vi "Automatic Teller Machine (ATM).vi"() -> ()   [LabVIEW 2013]
uses:
  Controls/ATM States.ctl
  Controls/Log Data States.ctl
  SubVIs/Function Command.ctl
  Controls/Function States.ctl
panel:
  in  "Enter":bool
  in  "User Input":string
  in  "Right Buttons":T1
  out "Right Menu":T2
  in  "Left Buttons":T1
  out "Left Menu":T2
  in  "Card Simulator":bool
  out "ATM Messages":string
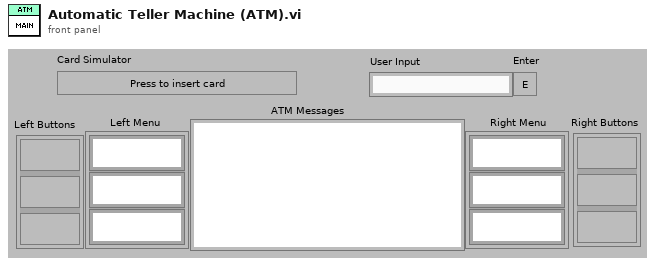
[diagram p1: front panel]
types:
  T1 = cluster{"Func Button":bool, "Func Button 2":bool, "Func Button 3":bool}
  T2 = cluster{"RFS String":string, "RFS String 2":string, "RFS String 3":string}
  T3 = cluster{"ATM Messages":string, "Left Menu":cluster{"RFS String":string, "RFS String 2":string, "RFS String 3":string}, "Right Menu":cluster{"RFS String":string, "RFS String 2":string, "RFS String 3":string}}
  T4 = typedef "ATM States.ctl" = enum16{"Initialize", "Account Check", "Main", "Withdraw", "Deposit", "Stop"}
  T5 = cluster{"Left Buttons":refnum<vi>, "Right Buttons":refnum<vi>, "Left Menu":refnum<vi>, "Right Menu":refnum<vi>, "User Input":refnum<vi>, "Enter":refnum<vi>}
  T6 = typedef "Function States.ctl" = enum16{"Check Account", "Deposit", "Withdraw"}
  T7 = typedef "Function Command.ctl" = enum16{"Set function", "Get function"}
  T8 = typedef "Log Data States.ctl" = enum16{"Initialize", "Read", "Write", "Stop"}
  T9 = enum8{"Enabled", "Disabled", "Disabled and Grayed Out"}
  T10 = cluster{"First Name":string, "Last Name":string, "Account No.":string, "Balance":i32}
  T11 = cluster{"First Name":string, "Last Name":string, "Account No.":string, "Balance":i32}[]
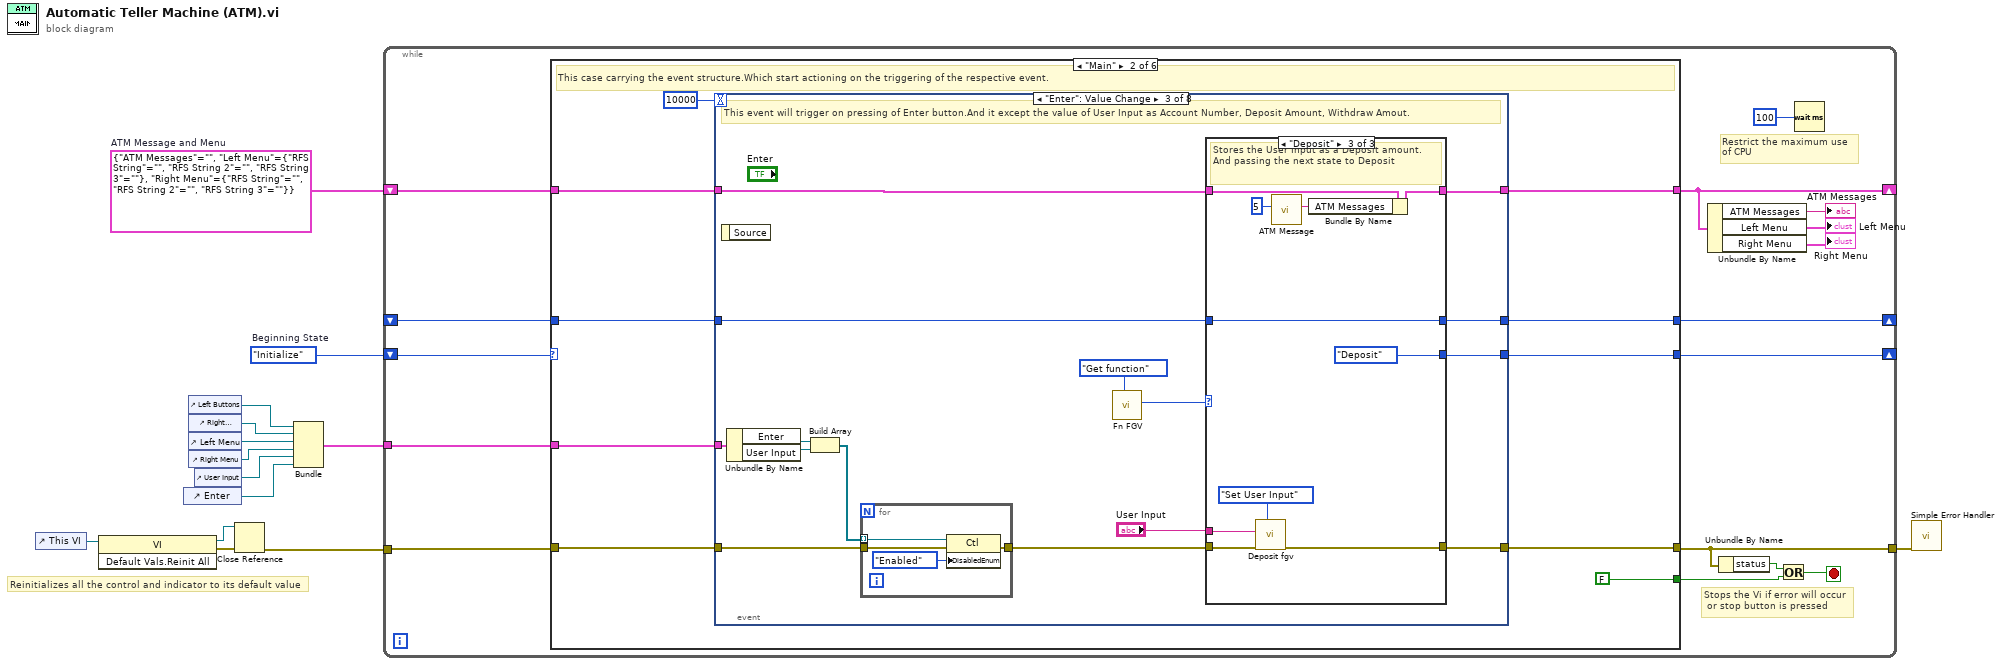
[diagram p0: block diagram]
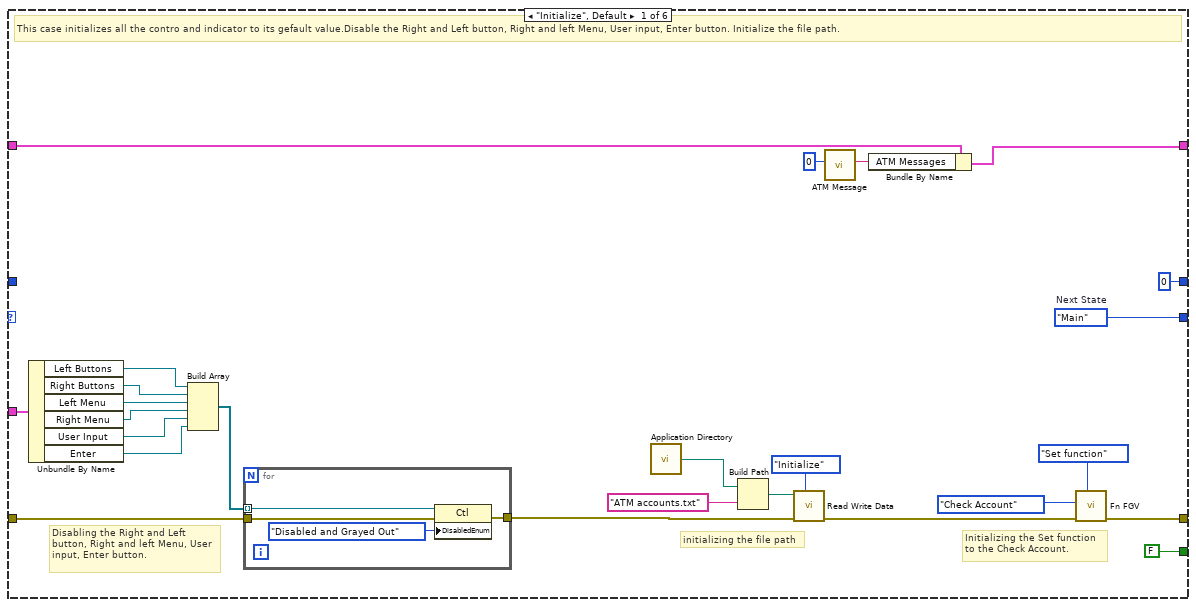
[diagram p2: hidden frame]
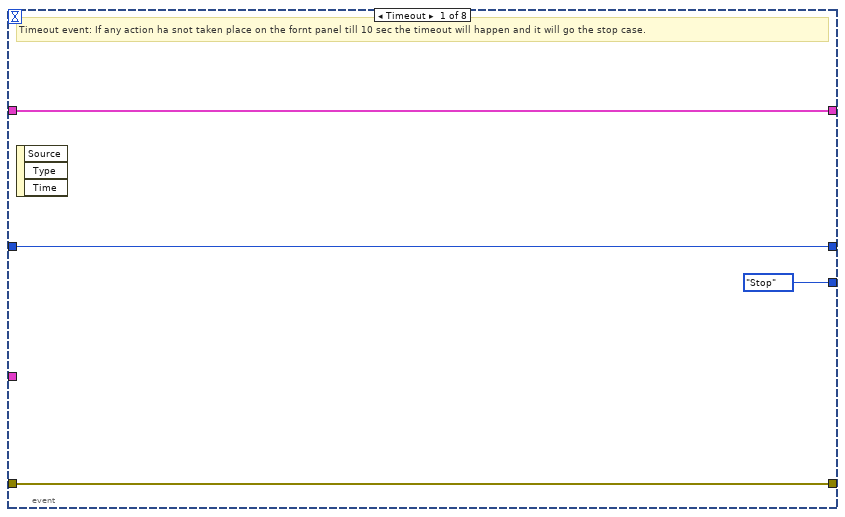
[diagram p3: hidden frame]
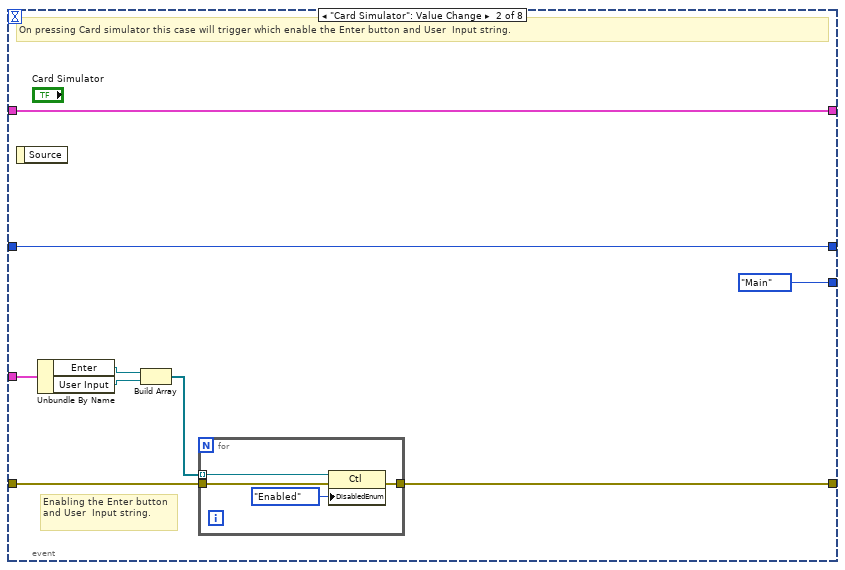
[diagram p4: hidden frame]
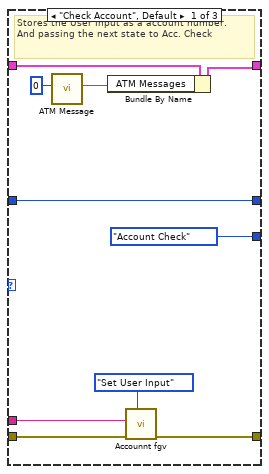
[diagram p5: hidden frame]
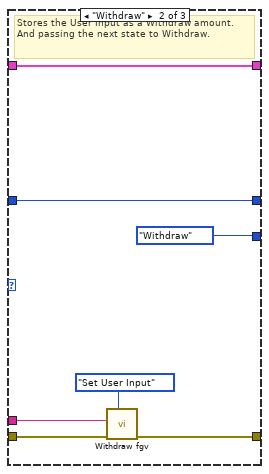
[diagram p6: hidden frame]
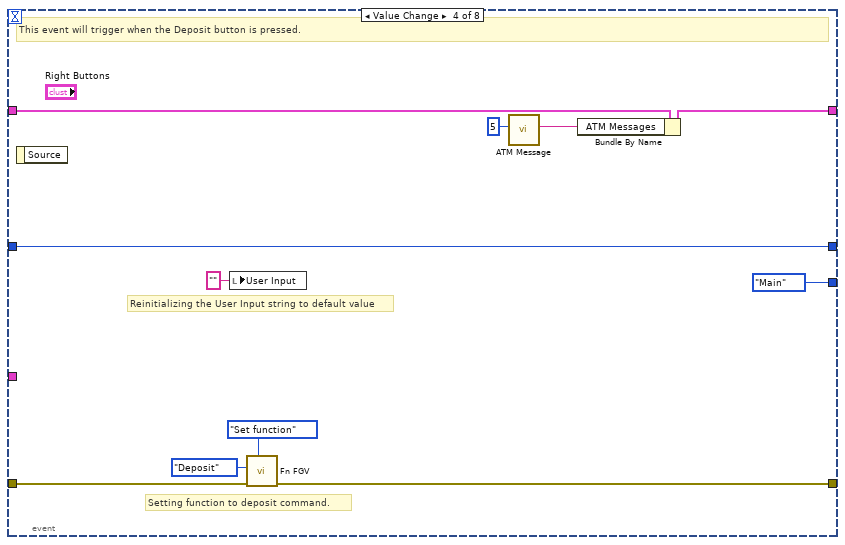
[diagram p7: hidden frame]
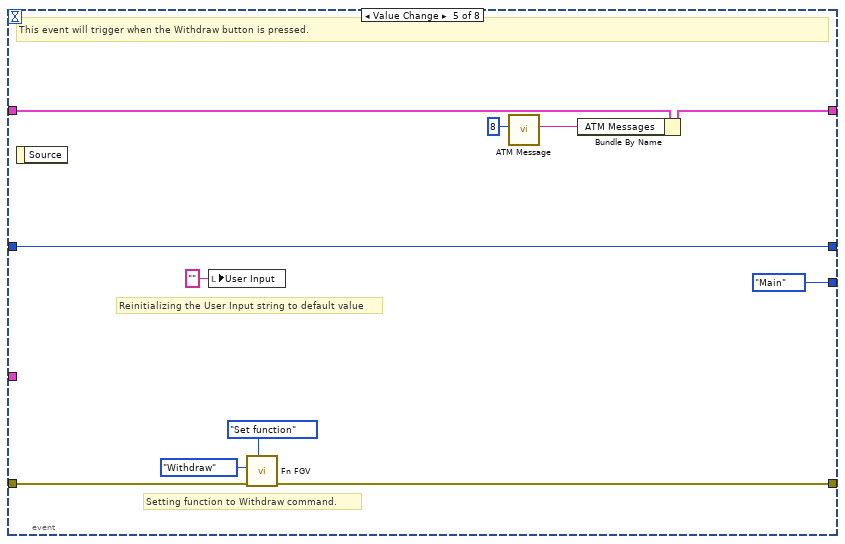
[diagram p8: hidden frame]
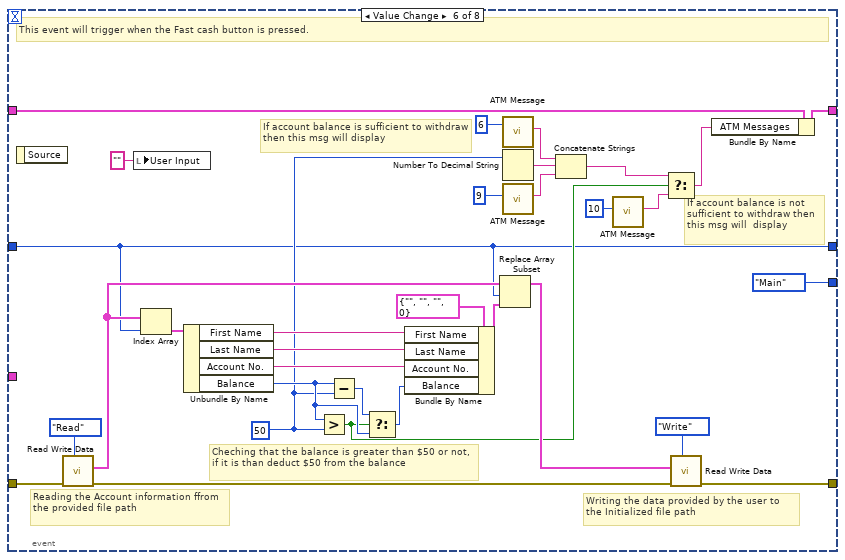
[diagram p9: hidden frame]
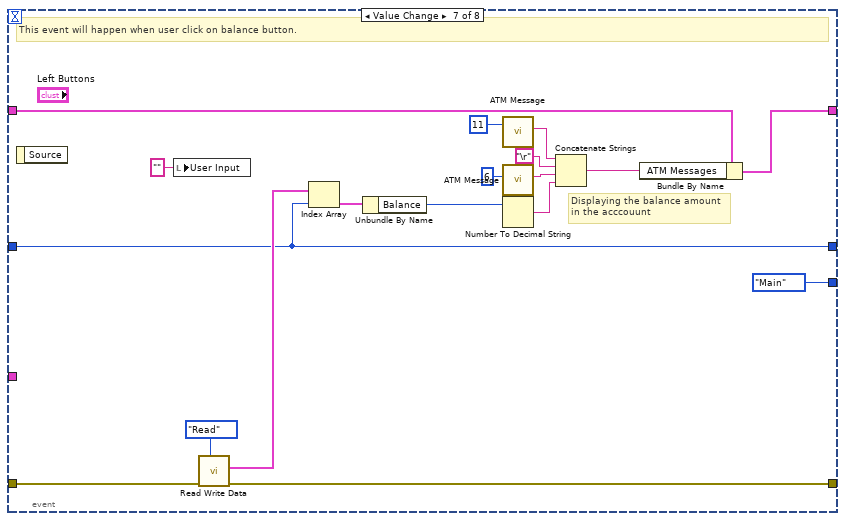
[diagram p10: hidden frame]
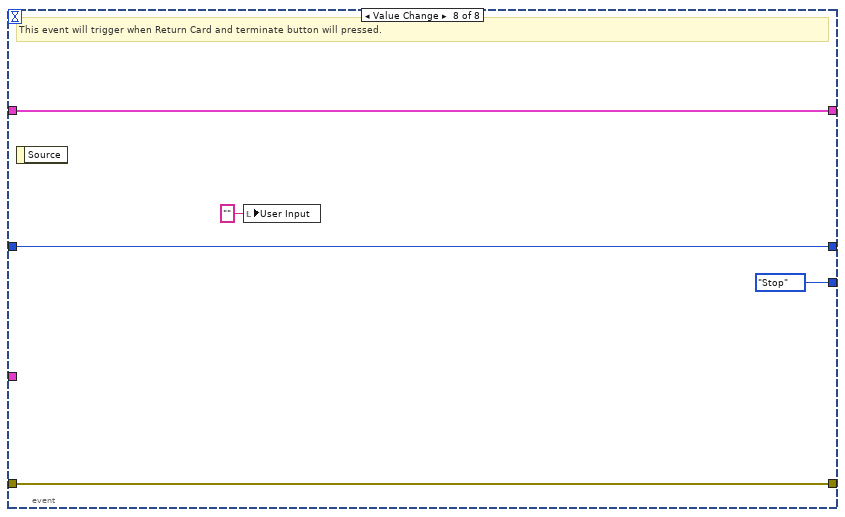
[diagram p11: hidden frame]
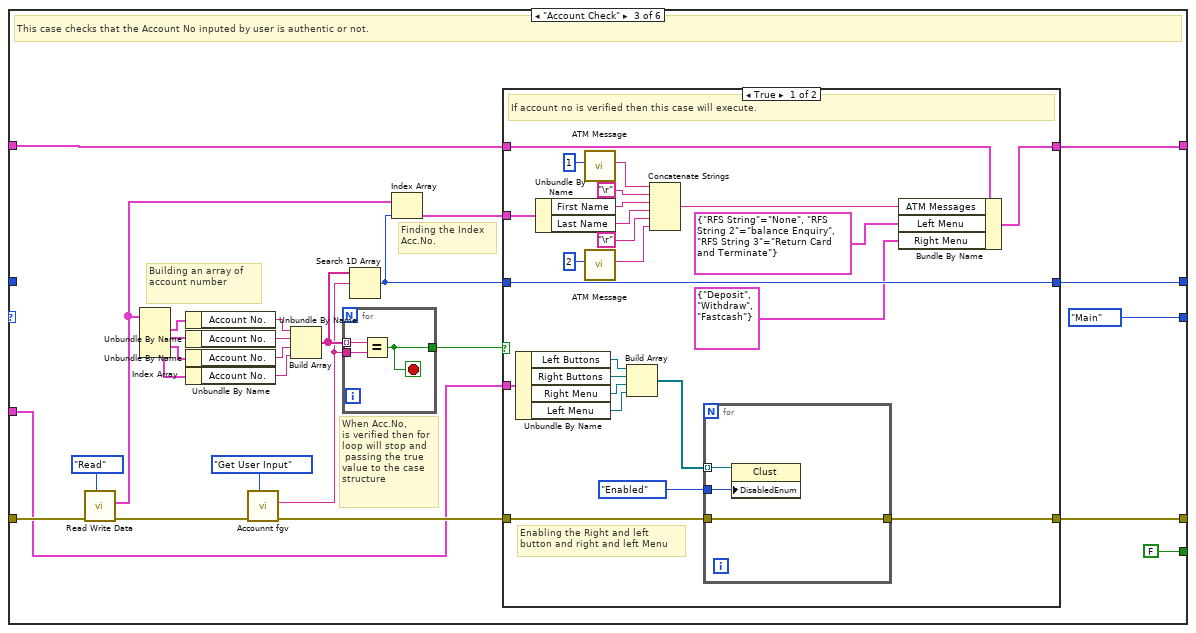
[diagram p12: hidden frame]
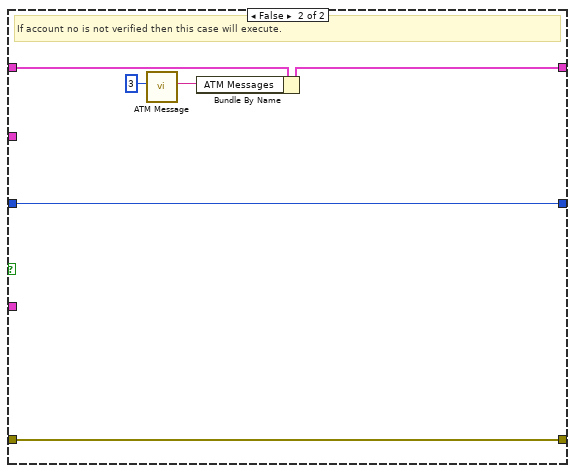
[diagram p13: hidden frame]
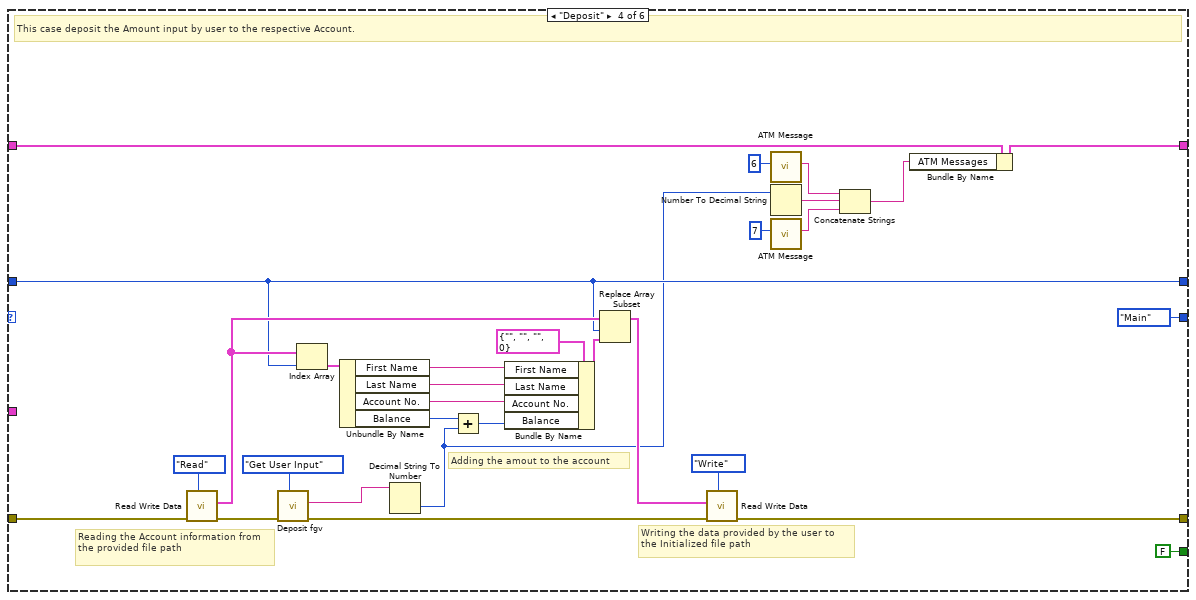
[diagram p14: hidden frame]
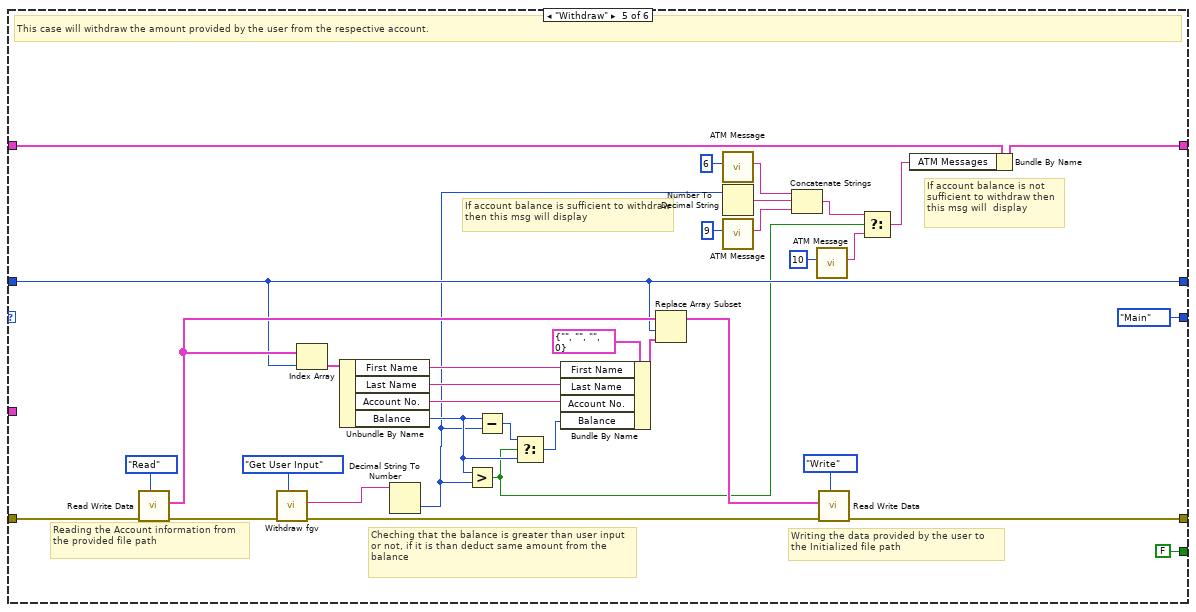
[diagram p15: hidden frame]
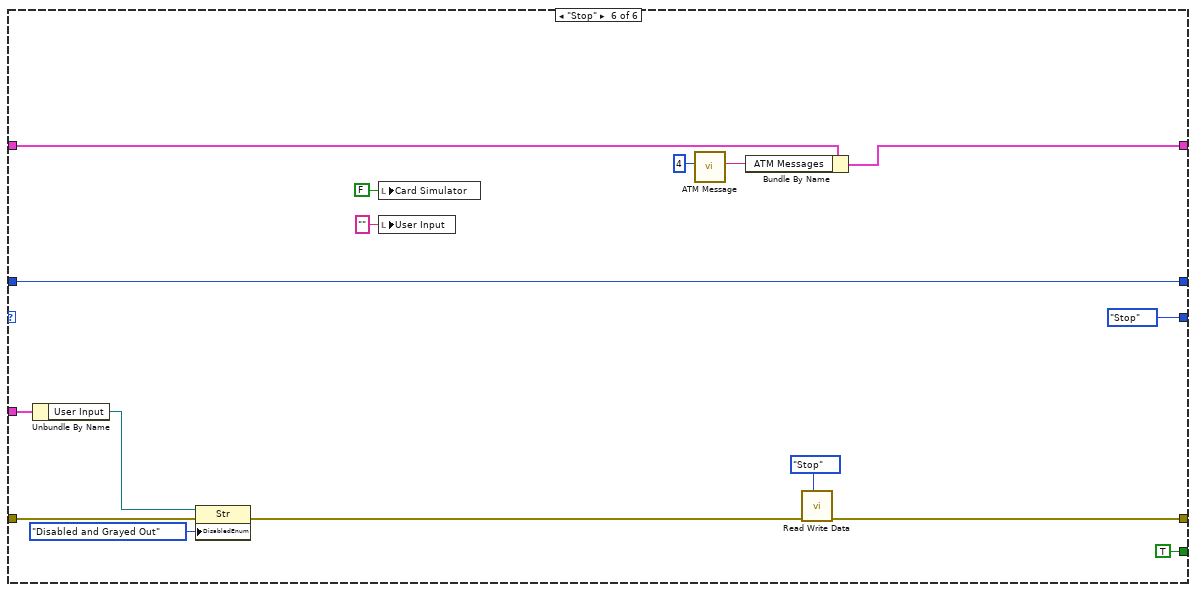
[diagram p16: hidden frame]
diagram:
  w1 = T3 {"ATM Messages"="", "Left Menu"={"RFS String"="", "RFS String 2"="", "RFS String 3"=""}, "Right Menu"={"RFS String"="", "RFS String 2"="", "RFS String 3"=""}}  # ATM Message and Menu
  w14 = ATM_States."Initialize"  # Beginning State
  # "Reinitializes all the control and indicator to its default value"
  n1 = control-ref of="This VI"() -> (w13:refnum<vi>)
  n2 = invoke class="VI" method="Default Vals.Reinit All"(reference=w13) -> (reference out=w11:refnum<vi>, error out=w12:errorcluster)  [unwired: 2 in, 1 out]
  n3 = control-ref of="Enter"() -> (w9:refnum<vi>)
  n4 = control-ref of="Left Buttons"() -> (w8:refnum<vi>)
  n5 = control-ref of="Right Buttons"() -> (w7:refnum<vi>)
  n6 = control-ref of="Left Menu"() -> (w6:refnum<vi>)
  n7 = control-ref of="Right Menu"() -> (w5:refnum<vi>)
  n8 = control-ref of="User Input"() -> (w4:refnum<vi>)
  n9 = Close Reference(reference=w11, error in (no error)=w12) -> (error out=w10:errorcluster)
  n10 = Bundle("Left Buttons"=w8, "Right Buttons"=w7, "Left Menu"=w6, "Right Menu"=w5, "User Input"=w4, "Enter"=w9) -> (w3:T5)  [unwired: 1 in]
  n11 = while {
    shift-right: [w29] -> _
    shift-left: w14 -> [w30]
    tunnel: w10 -> [w27]
    tunnel: [w26] -> w2
    tunnel: w3 -> [w22]
    shift-right: [w20] -> _
    shift-left: w1 -> [w21]
    shift-right: [w16] -> _
    shift-left: _ -> [w15]
    stop <- w24 stop-if-true
    # "Restrict the maximum use \nof CPU"
    # "Stops the Vi if error will occur\n or stop button is pressed"
    n12 = case shown="\"Main\"" w30 {
      tunnel: [w55 w66 ATM_States."Main" ("Next State") ATM_States."Main" ("Next State") ATM_States."Main" ("Next State") ATM_States."Stop" ("Next State")] -> w29
      tunnel: w27 -> [w45 w69 w216 w296 w333 w342]
      tunnel: [w38 w68 w212 w300 w335 w338] -> w26
      tunnel: [FALSE FALSE FALSE FALSE FALSE TRUE] -> w23
      tunnel: [w35 w64 w210 w284 w323 w348] -> w20
      tunnel: w22 -> [w53 w62 w214 _ _ w344]
      tunnel: w21 -> [w36 w63 w215 w301 w336 w349]
      tunnel: [0 ("index of element") w60 w213 w275 w317 w345] -> w16
      tunnel: w15 -> [_ w61 _ w275 w317 w345]
      frame "Initialize", Default {
        w55 = ATM_States."Main"  # Next State
        # "Initializing the Set function\nto the Check Account."
        # "initializing the file path"
        # "Disabling the Right and Left button, Right and left Menu, User input, Enter button."
        # "This case initializes all the contro and indicator to its gefault value.Disable the Right and Left button, Right and left Menu, User input, Enter button. Initialize the file path."
        n13 = Unbundle By Name(w53) -> ("Left Buttons"=w52:refnum<vi>, "Right Buttons"=w51:refnum<vi>, "Left Menu"=w50:refnum<vi>, "Right Menu"=w49:refnum<vi>, "User Input"=w48:refnum<vi>, "Enter"=w47:refnum<vi>)
        n14 = Build Array(w52, w51, w50, w49, w48, w47) -> (w46:refnum<vi>[])
        n15 = for {
          tunnel: w46 -> [w59] mode=indexing
          tunnel: w45 -> [w57]
          tunnel: [w56] -> w44
          n16 = property on="Property Node" class="Ctl"(reference=w59, error in=w57, "DisabledEnum"=T9."Disabled and Grayed Out" ("Disabled")) -> (error out=w56:errorcluster)  [unwired: 1 out]
        }
        n17 = call <vilib>:"Application Directory.vi"() -> ("Application Directory"=w42:path)
        n18 = Build Path(base path=w42, name or relative path="ATM accounts.txt") -> (appended path=w40:path)
        n19 = call "Read Write Data.vi"("Enum"=Log_Data_States."Initialize", "error in (no error)"=w44, "file path"=w40) -> ("error out"=w39:errorcluster)  [unwired: 7 in, 1 out]
        n20 = call "ATM Message.vi"("Index"=0) -> ("Message"=w34:string)  [unwired: 9 in, 1 out]
        n21 = Bundle By Name(cluster=w36, "ATM Messages"=w34) -> (w35:T3)
        n22 = call "Fn FGV.vi"("Command"=Function_Command."Set function", "error in (no error)"=w39, "Enum in"=Function_States."Check Account") -> ("error out"=w38:errorcluster)  [unwired: 7 in, 1 out]
      }
      frame "Main" {
        # "This case carrying the event structure.Which start actioning on the triggering of the respective event."
        n23 = event shown="[2] \"Enter\": Value Change" {
          selector: _ -> [_ _ _ _ _ _ _ _]
          dyn-events: _ -> [_ _ _ _ _ _ _ _]
          timeout: 10000 -> [_ _ _ _ _ _ _ _]
          tunnel: w69 -> [w73 w78 w89 w140 w151 w160 w195 w209]
          tunnel: [w73 w77 w91 w139 w150 w159 w196 w209] -> w68
          tunnel: [ATM_States."Stop" ("Beginning State") ATM_States."Main" ("Beginning State") w92 ATM_States."Main" ("Beginning State") ATM_States."Main" ("Beginning State") ATM_States."Main" ("Beginning State") ATM_States."Main" ("Beginning State") ATM_States."Stop" ("Beginning State")] -> w66
          tunnel: w62 -> [_ w82 w101 _ _ _ _ _]
          tunnel: [w71 w76 w93 w136 w147 w157 w193 w208] -> w64
          tunnel: w63 -> [w71 w76 w94 w143 w154 w186 w204 w208]
          tunnel: w61 -> [w70 w74 w88 w133 w144 w155 w187 w205]
          tunnel: [w70 w74 w87 w133 w144 w155 w187 w205] -> w60
          event Timeout {
            # "Timeout event: If any action ha snot taken place on the fornt panel till 10 sec the timeout will happen and it will go the stop case."
            n24 = event-data() -> ()  [unwired: 1 in, 3 out]
          }
          event "Card Simulator": Value Change {
            # "Enabling the Enter button and User  Input string."
            # "On pressing Card simulator this case will trigger which enable the Enter button and User  Input string."
            n25 = event-data() -> ()  [unwired: 1 in, 1 out]
            n26 = Unbundle By Name(w82) -> ("Enter"=w81:refnum<vi>, "User Input"=w80:refnum<vi>)
            n27 = Build Array(w81, w80) -> (w79:refnum<vi>[])
            n28 = for {
              tunnel: w79 -> [w86] mode=indexing
              tunnel: w78 -> [w85]
              tunnel: [w84] -> w77
              n29 = property class="Ctl"(reference=w86, error in=w85, "DisabledEnum"=T9."Enabled" ("Disabled")) -> (error out=w84:errorcluster)  [unwired: 1 out]
            }
          }
          event "Enter": Value Change {
            # "This event will trigger on pressing of Enter button.And it except the value of User Input as Account Number, Deposit Amount, Withdraw Amout."
            n30 = event-data() -> ()  [unwired: 1 in, 1 out]
            n31 = Unbundle By Name(w101) -> ("Enter"=w100:refnum<vi>, "User Input"=w99:refnum<vi>)
            n32 = Build Array(w100, w99) -> (w98:refnum<vi>[])
            n33 = for {
              tunnel: w98 -> [w132] mode=indexing
              tunnel: w89 -> [w131]
              tunnel: [w130] -> w95
              n34 = property class="Ctl"(reference=w132, error in=w131, "DisabledEnum"=T9."Enabled" ("Disabled")) -> (error out=w130:errorcluster)  [unwired: 1 out]
            }
            n35 = call "Fn FGV.vi"("Command"=Function_Command."Get function") -> ("Enum out"=w97:T6)  [unwired: 9 in, 1 out]
            n36 = case shown="\"Deposit\"" w97 {
              tunnel: "User Input" -> [w110 w116 w128]
              tunnel: w95 -> [w111 w118 w127]
              tunnel: [w107 w114 w124] -> w91
              tunnel: [ATM_States."Account Check" ("Beginning State") ATM_States."Withdraw" ("Beginning State") ATM_States."Deposit" ("Beginning State")] -> w92
              tunnel: [w104 w113 w122] -> w93
              tunnel: w94 -> [w105 w113 w123]
              tunnel: w88 -> [w102 w112 w119]
              tunnel: [w102 w112 w119] -> w87
              frame "Check Account", Default {
                # "Stores the User Input as a account number.\nAnd passing the next state to Acc. Check"
                n37 = call "ATM Message.vi"("Index"=0) -> ("Message"=w103:string)  [unwired: 9 in, 1 out]
                n38 = Bundle By Name(cluster=w105, "ATM Messages"=w103) -> (w104:T3)
                n39 = call "Accounnt fgv.vi"("Command"=enum16{"Set User Input", "Get User Input"}."Set User Input", "error in (no error)"=w111, "User Input IN"=w110) -> ("error out"=w107:errorcluster)  [unwired: 7 in, 1 out]
              }
              frame "Withdraw" {
                # "Stores the User Input as a Withdraw amount.\nAnd passing the next state to Withdraw."
                n40 = call "Withdraw fgv.vi"("Command"=enum16{"Set User Input", "Get User Input"}."Set User Input", "error in (no error)"=w118, "User Input IN  in"=w116) -> ("error out"=w114:errorcluster)  [unwired: 7 in, 1 out]
              }
              frame "Deposit" {
                # "Stores the User Input as a Deposit amount.\nAnd passing the next state to Deposit"
                n41 = call "Deposit fgv.vi"("Command"=enum16{"Set User Input", "Get User Input"}."Set User Input", "error in (no error)"=w127, "User Input IN  in"=w128) -> ("error out"=w124:errorcluster)  [unwired: 7 in, 1 out]
                n42 = call "ATM Message.vi"("Index"=5) -> ("Message"=w121:string)  [unwired: 9 in, 1 out]
                n43 = Bundle By Name(cluster=w123, "ATM Messages"=w121) -> (w122:T3)
              }
            }
          }
          event "Right Buttons.Func Button": Value Change {
            # "Reinitializing the User Input string to default value"
            # "Setting function to deposit command."
            # "This event will trigger when the Deposit button is pressed."
            n44 = event-data() -> ()  [unwired: 1 in, 1 out]
            n45 = local write "User Input"("" ("User Input")) -> ()
            n46 = call "Fn FGV.vi"("Command"=Function_Command."Set function", "error in (no error)"=w140, "Enum in"=Function_States."Deposit") -> ("error out"=w139:errorcluster)  [unwired: 7 in, 1 out]
            n47 = call "ATM Message.vi"("Index"=5) -> ("Message"=w135:string)  [unwired: 9 in, 1 out]
            n48 = Bundle By Name(cluster=w143, "ATM Messages"=w135) -> (w136:T3)
          }
          event "Right Buttons.Func Button 2": Value Change {
            # "Setting function to Withdraw command."
            # "Reinitializing the User Input string to default value"
            # "This event will trigger when the Withdraw button is pressed."
            n49 = event-data() -> ()  [unwired: 1 in, 1 out]
            n50 = local write "User Input"("" ("User Input")) -> ()
            n51 = call "Fn FGV.vi"("Command"=Function_Command."Set function", "error in (no error)"=w151, "Enum in"=Function_States."Withdraw") -> ("error out"=w150:errorcluster)  [unwired: 7 in, 1 out]
            n52 = call "ATM Message.vi"("Index"=8) -> ("Message"=w146:string)  [unwired: 9 in, 1 out]
            n53 = Bundle By Name(cluster=w154, "ATM Messages"=w146) -> (w147:T3)
          }
          event "Right Buttons.Func Button 3": Value Change {
            w161 = 50
            # "If account balance is not sufficient to withdraw then this msg will  display"
            # "If account balance is sufficient to withdraw then this msg will display"
            # "Writing the data provided by the user to the Initialized file path"
            # "Cheching that the balance is greater than $50 or not, if it is than deduct $50 from the balance"
            # "Reading the Account information ffrom the provided file path"
            # "This event will trigger when the Fast cash button is pressed."
            n54 = event-data() -> ()  [unwired: 1 in, 1 out]
            n55 = call "Read Write Data.vi"("Enum"=Log_Data_States."Read", "error in (no error)"=w160) -> ("error out"=w162:errorcluster, "Array"=w180:T11)  [unwired: 8 in]
            n56 = local write "User Input"("" ("User Input")) -> ()
            n57 = Index Array(array=w180, index=w155) -> (element=w179:T10)
            n58 = Unbundle By Name(w179) -> ("First Name"=w178:string, "Last Name"=w177:string, "Account No."=w176:string, "Balance"=w167:i32)
            n59 = Greater?(x=w167, y=w161) -> (0:w163:bool)
            n60 = Subtract(x=w167, y=w161) -> (x-y=w169:i32)
            n61 = Select(t=w169, s=w163, f=w167) -> (s? t:f=w168:i32)
            n62 = Bundle By Name(cluster=T10 {"First Name"="", "Last Name"="", "Account No."="", "Balance"=0}, "First Name"=w178, "Last Name"=w177, "Account No."=w176, "Balance"=w168) -> (w181:T10)
            n63 = Replace Array Subset(array=w180, new element=w181, index=w155) -> (w175:T11)
            n64 = call "ATM Message.vi"("Index"=6) -> ("Message"=w172:string)  [unwired: 9 in, 1 out]
            n65 = Number To Decimal String(number=w161) -> (decimal integer string=w171:string)  [unwired: 1 in]
            n66 = call "ATM Message.vi"("Index"=9) -> ("Message"=w170:string)  [unwired: 9 in, 1 out]
            n67 = Concatenate Strings(w172, w171, w170) -> (w164:string)
            n68 = call "ATM Message.vi"("Index"=10) -> ("Message"=w165:string)  [unwired: 9 in, 1 out]
            n69 = Select(t=w164, s=w163, f=w165) -> (s? t:f=w156:string)
            n70 = call "Read Write Data.vi"("Enum"=Log_Data_States."Write", "error in (no error)"=w162, "Account Information"=w175) -> ("error out"=w159:errorcluster)  [unwired: 7 in, 1 out]
            n71 = Bundle By Name(cluster=w186, "ATM Messages"=w156) -> (w157:T3)
          }
          event "Left Buttons.Func Button 2": Value Change {
            # "Displaying the balance amount in the acccouunt"
            # "This event will happen when user click on balance button."
            n72 = event-data() -> ()  [unwired: 1 in, 1 out]
            n73 = local write "User Input"("" ("User Input")) -> ()
            n74 = call "Read Write Data.vi"("Enum"=Log_Data_States."Read", "error in (no error)"=w195) -> ("error out"=w196:errorcluster, "Array"=w201:T11)  [unwired: 8 in]
            n75 = Index Array(array=w201, index=w187) -> (element=w200:T10)
            n76 = Unbundle By Name(w200) -> ("Balance"=w190:i32)
            n77 = call "ATM Message.vi"("Index"=11) -> ("Message"=w198:string)  [unwired: 9 in, 1 out]
            n78 = call "ATM Message.vi"("Index"=6) -> ("Message"=w189:string)  [unwired: 9 in, 1 out]
            n79 = Number To Decimal String(number=w190) -> (decimal integer string=w188:string)  [unwired: 1 in]
            n80 = Concatenate Strings(w198, "\r", w189, w188) -> (w197:string)
            n81 = Bundle By Name(cluster=w204, "ATM Messages"=w197) -> (w193:T3)
          }
          event "Left Buttons.Func Button 3": Value Change {
            # "This event will trigger when Return Card and terminate button will pressed."
            n82 = event-data() -> ()  [unwired: 1 in, 1 out]
            n83 = local write "User Input"("" ("User Input")) -> ()
          }
        }
      }
      frame "Account Check" {
        # "Finding the Index \nAcc.No."
        # "When Acc.No,\nis verified then for\nloop will stop and\n passing the true \nvalue to the case \nstructure"
        # "Building an array of account number"
        # "This case checks that the Account No inputed by user is authentic or not."
        n84 = call "Read Write Data.vi"("Enum"=Log_Data_States."Read", "error in (no error)"=w216) -> ("error out"=w224:errorcluster, "Array"=w219:T11)  [unwired: 8 in]
        n85 = Index Array(array=w219) -> (element #1=w232:T10, element #2=w231:T10, element #3=w230:T10, element #4=w229:T10)  [unwired: 4 in]
        n86 = Unbundle By Name(w232) -> ("Account No."=w228:string)
        n87 = Unbundle By Name(w231) -> ("Account No."=w227:string)
        n88 = Unbundle By Name(w230) -> ("Account No."=w226:string)
        n89 = Unbundle By Name(w229) -> ("Account No."=w225:string)
        n90 = call "Accounnt fgv.vi"("Command"=enum16{"Set User Input", "Get User Input"}."Get User Input", "error in (no error)"=w224) -> ("error out"=w217:errorcluster, "User Input OUT"=w221:string)  [unwired: 8 in]
        n91 = Build Array(w228, w227, w226, w225) -> (w222:string[])
        n92 = for {
          tunnel: w222 -> [w271] mode=indexing
          tunnel: w221 -> [w270]
          tunnel: [w269] -> w223
          stop <- w269 stop-if-true
          n93 = Equal?(x=w271, y=w270) -> (x = y?=w269:bool)
        }
        n94 = Search 1D Array(1D array=w222, element=w221) -> (index of element=w220:i32)  [unwired: 1 in]
        n95 = Index Array(array=w219, index=w220) -> (element=w218:T10)
        n96 = case shown="True" w223 {
          tunnel: w215 -> [w259 w268]
          tunnel: [w258 w267] -> w210
          tunnel: [w256 w265] -> w213
          tunnel: w220 -> [w256 w265]
          tunnel: w218 -> [w255 _]
          tunnel: w217 -> [w239 w263]
          tunnel: [w238 w263] -> w212
          tunnel: w214 -> [w246 _]
          frame True {
            # "Enabling the Right and left \nbutton and right and left Menu"
            # "If account no is verified then this case will execute."
            n97 = Unbundle By Name(w246) -> ("Left Buttons"=w245:refnum<vi>, "Right Buttons"=w242:refnum<vi>, "Right Menu"=w243:refnum<vi>, "Left Menu"=w244:refnum<vi>)
            n98 = Unbundle By Name(w255) -> ("First Name"=w249:string, "Last Name"=w250:string)
            n99 = call "ATM Message.vi"("Index"=1) -> ("Message"=w253:string)  [unwired: 9 in, 1 out]
            n100 = call "ATM Message.vi"("Index"=2) -> ("Message"=w251:string)  [unwired: 9 in, 1 out]
            n101 = Build Array(w245, w242, w243, w244) -> (w240:refnum<vi>[])
            n102 = Concatenate Strings(w253, "\r", w249, w250, "\r", w251) -> (w252:string)
            n103 = for {
              tunnel: T9."Enabled" ("Disabled") -> [w262]
              tunnel: w240 -> [w261] mode=indexing
              tunnel: w239 -> [w260]
              tunnel: [w260] -> w238
              n104 = property class="Clust"(reference=w261, "DisabledEnum"=w262) -> ()  [unwired: 1 in, 2 out]
            }
            n105 = Bundle By Name(cluster=w259, "ATM Messages"=w252, "Left Menu"=T2 {"RFS String"="None", "RFS String 2"="balance Enquiry", "RFS String 3"="Return Card and Terminate"}, "Right Menu"=T2 {"RFS String"="Deposit", "RFS String 2"="Withdraw", "RFS String 3"="Fastcash"}) -> (w258:T3)
          }
          frame False {
            # "If account no is not verified then this case will execute."
            n106 = call "ATM Message.vi"("Index"=3) -> ("Message"=w264:string)  [unwired: 9 in, 1 out]
            n107 = Bundle By Name(cluster=w268, "ATM Messages"=w264) -> (w267:T3)
          }
        }
      }
      frame "Deposit" {
        # "Adding the amout to the account"
        # "Reading the Account information from the provided file path"
        # "Writing the data provided by the user to the Initialized file path"
        # "This case deposit the Amount input by user to the respective Account."
        n108 = call "Read Write Data.vi"("Enum"=Log_Data_States."Read", "error in (no error)"=w296) -> ("error out"=w295:errorcluster, "Array"=w291:T11)  [unwired: 8 in]
        n109 = call "Deposit fgv.vi"("Command"=enum16{"Set User Input", "Get User Input"}."Get User Input", "error in (no error)"=w295) -> ("error out"=w298:errorcluster, "User Input IN  out"=w286:string)  [unwired: 8 in]
        n110 = Index Array(array=w291, index=w275) -> (element=w290:T10)
        n111 = Unbundle By Name(w290) -> ("First Name"=w289:string, "Last Name"=w288:string, "Account No."=w287:string, "Balance"=w281:i32)
        n112 = Decimal String To Number(string=w286) -> (number=w273:i32)  [unwired: 2 in, 1 out]
        n113 = Add(x=w281, y=w273) -> (x+y=w280:i32)
        n114 = Bundle By Name(cluster=T10 {"First Name"="", "Last Name"="", "Account No."="", "Balance"=0}, "First Name"=w289, "Last Name"=w288, "Account No."=w287, "Balance"=w280) -> (w292:T10)
        n115 = Replace Array Subset(array=w291, new element=w292, index=w275) -> (w285:T11)
        n116 = call "Read Write Data.vi"("Enum"=Log_Data_States."Write", "error in (no error)"=w298, "Account Information"=w285) -> ("error out"=w300:errorcluster)  [unwired: 7 in, 1 out]
        n117 = call "ATM Message.vi"("Index"=6) -> ("Message"=w279:string)  [unwired: 9 in, 1 out]
        n118 = Number To Decimal String(number=w273) -> (decimal integer string=w278:string)  [unwired: 1 in]
        n119 = call "ATM Message.vi"("Index"=7) -> ("Message"=w277:string)  [unwired: 9 in, 1 out]
        n120 = Concatenate Strings(w279, w278, w277) -> (w276:string)
        n121 = Bundle By Name(cluster=w301, "ATM Messages"=w276) -> (w284:T3)
      }
      frame "Withdraw" {
        # "If account balance is not sufficient to withdraw then this msg will  display"
        # "Writing the data provided by the user to the Initialized file path"
        # "If account balance is sufficient to withdraw then this msg will display"
        # "Cheching that the balance is greater than user input or not, if it is than deduct same amount from the balance"
        # "Reading the Account information from the provided file path"
        # "This case will withdraw the amount provided by the user from the respective account."
        n122 = call "Read Write Data.vi"("Enum"=Log_Data_States."Read", "error in (no error)"=w333) -> ("error out"=w306:errorcluster, "Array"=w329:T11)  [unwired: 8 in]
        n123 = call "Withdraw fgv.vi"("Command"=enum16{"Set User Input", "Get User Input"}."Get User Input", "error in (no error)"=w306) -> ("error out"=w305:errorcluster, "User Input IN  out"=w304:string)  [unwired: 8 in]
        n124 = Index Array(array=w329, index=w317) -> (element=w328:T10)
        n125 = Unbundle By Name(w328) -> ("First Name"=w327:string, "Last Name"=w326:string, "Account No."=w325:string, "Balance"=w313:i32)
        n126 = Decimal String To Number(string=w304) -> (number=w307:i32)  [unwired: 2 in, 1 out]
        n127 = Greater?(x=w313, y=w307) -> (0:w309:bool)
        n128 = Subtract(x=w313, y=w307) -> (x-y=w315:i32)
        n129 = Select(t=w315, s=w309, f=w313) -> (s? t:f=w314:i32)
        n130 = Bundle By Name(cluster=T10 {"First Name"="", "Last Name"="", "Account No."="", "Balance"=0}, "First Name"=w327, "Last Name"=w326, "Account No."=w325, "Balance"=w314) -> (w330:T10)
        n131 = Replace Array Subset(array=w329, new element=w330, index=w317) -> (w324:T11)
        n132 = call "ATM Message.vi"("Index"=6) -> ("Message"=w320:string)  [unwired: 9 in, 1 out]
        n133 = Number To Decimal String(number=w307) -> (decimal integer string=w319:string)  [unwired: 1 in]
        n134 = call "ATM Message.vi"("Index"=9) -> ("Message"=w318:string)  [unwired: 9 in, 1 out]
        n135 = Concatenate Strings(w320, w319, w318) -> (w310:string)
        n136 = call "ATM Message.vi"("Index"=10) -> ("Message"=w311:string)  [unwired: 9 in, 1 out]
        n137 = call "Read Write Data.vi"("Enum"=Log_Data_States."Write", "error in (no error)"=w305, "Account Information"=w324) -> ("error out"=w335:errorcluster)  [unwired: 7 in, 1 out]
        n138 = Select(t=w310, s=w309, f=w311) -> (s? t:f=w308:string)
        n139 = Bundle By Name(cluster=w336, "ATM Messages"=w308) -> (w323:T3)
      }
      frame "Stop" {
        n140 = Unbundle By Name(w344) -> ("User Input"=w343:refnum<vi>)
        n141 = property on="Property Node" class="Str"(reference=w343, error in=w342, "DisabledEnum"=T9."Disabled and Grayed Out" ("Disabled")) -> (error out=w339:errorcluster)  [unwired: 1 out]
        n142 = local write "Card Simulator"(FALSE ("Card Simulator")) -> ()
        n143 = local write "User Input"("" ("User Input")) -> ()
        n144 = call "ATM Message.vi"("Index"=4) -> ("Message"=w351:string)  [unwired: 9 in, 1 out]
        n145 = Bundle By Name(cluster=w349, "ATM Messages"=w351) -> (w348:T3)
        n146 = call "Read Write Data.vi"("Enum"=Log_Data_States."Stop", "error in (no error)"=w339) -> ("error out"=w338:errorcluster)  [unwired: 8 in, 1 out]
      }
    }
    n147 = Unbundle By Name(w20) -> ("ATM Messages"=→"ATM Messages":string, "Left Menu"=→"Left Menu":T2, "Right Menu"=→"Right Menu":T2)
    n148 = Unbundle By Name(w26) -> ("status"=w25:bool)
    n149 = Or(x=w25, y=w23) -> (x .or. y?=w24:bool)
    n150 = Wait (ms)(milliseconds to wait=u32 100) -> ()  [unwired: 1 out]
  }
  n151 = call <vilib>:"Simple Error Handler.vi"("error in (no error)"=w2) -> ()  [unwired: 4 in, 5 out]
